vi "Test Flatten.vi"() -> ()   [LabVIEW 2021]
uses:
  CIFfifo.lvclass
  CIFfifo.lvclass/CIFfifo.ctl
  Utilities/Unflatten FIFO Config.vi
  Accessors/Write Header.vi
  Accessors/Write Flags.vi
  Accessors/Write ClockID.vi
  Accessors/Write Buffer.vi
  <vilib>/CIF Foundation/CIF Utilities/DataTypes/Unflatten U64.vi
  Utilities/Expand FIFO Flags.vi
  <userlib>/_OpenG.lib/numeric/numeric.llb/Random Number Within Range - DBL__ogtk.vi
  <userlib>/_OpenG.lib/numeric/numeric.llb/openg_numeric__ogtk.lvlib
panel:
  out "Input":u8[](array[numeric]) format="%.0x"
  out "Output":u8[](array[numeric]) format="%.0x"
  out "pass":bool
  out "error out":errorcluster
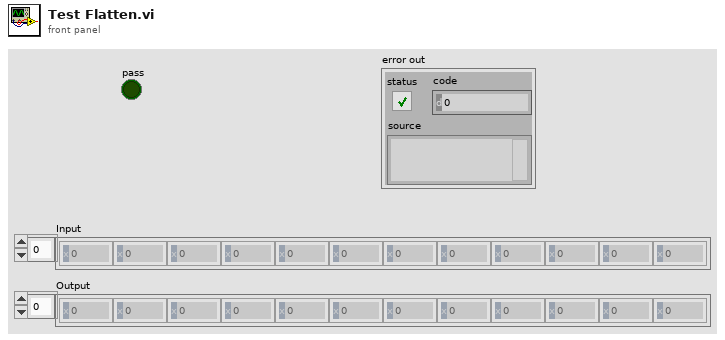
[diagram p1: front panel]
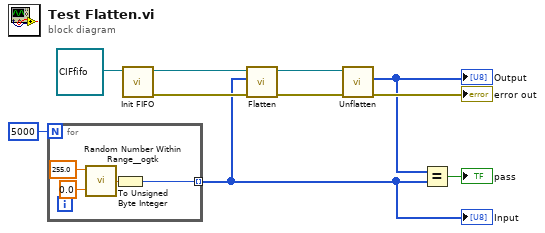
[diagram p0: block diagram]
diagram:
  n1 = for {
    N: 5000 -> [_]
    tunnel: [w11] -> w3 mode=indexing
    n2 = call-poly <userlib>:"Random Number Within Range__ogtk.vi"("High"=255.0, "Low"=0.0) -> ("Random Number"=w12:dbl)  [unwired: 3 in]
    n3 = To Unsigned Byte Integer(number=w12) -> (unsigned 8bit integer=w11:u8)
  }
  "Input" <- w3
  n4 = call "Init FIFO.vi"("CIFfifo in"=refnum<class "CIFfifo.lvclass"> refnum) -> ("error out"=w7:errorcluster, "CIFfifo out"=w9:refnum<class "CIFfifo.lvclass">)  [unwired: 8 in, 1 out]
  n5 = call "Flatten.vi"("error in (no error)"=w7, "Data in"=w3, "CIFfifo in"=w9) -> ("error out"=w8:errorcluster, "CIFfifo out"=w10:refnum<class "CIFfifo.lvclass">)  [unwired: 7 in]
  n6 = call "Unflatten.vi"("error in (no error)"=w8, "CIFfifo in"=w10) -> ("error out"=→"error out":errorcluster, "Data"=w4:u8[])  [unwired: 6 in, 2 out]
  "Output" <- w4
  n7 = Equal?(x=w4, y=w3) -> (x = y?=→"pass":bool)
